vi "While_For_DIsplay-MSI.vi"() -> ()   [LabVIEW 2020]
panel:
  out "e 2":bool
  out "f 2":bool
  out "g 2":bool
  out "d 2":bool
  out "c 2":bool
  out "b 2":bool
  out "a 2":bool
  in  "stop":bool
  out "a":bool
  out "b":bool
  out "c":bool
  out "d":bool
  out "g":bool
  out "f":bool
  out "e":bool
  # "While"
  # "For"
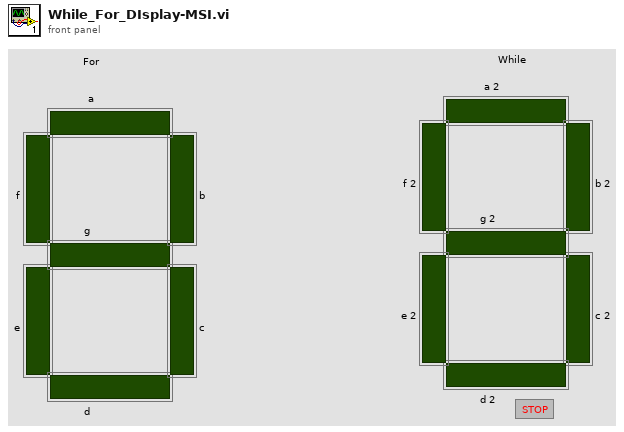
[diagram p1: front panel]
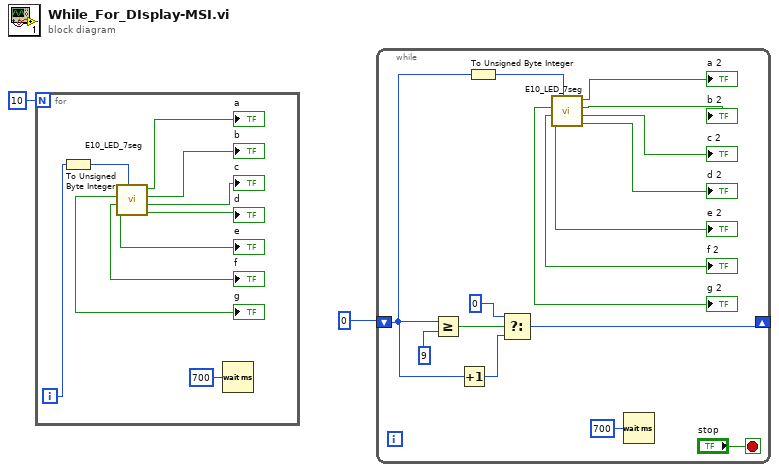
[diagram p0: block diagram]
diagram:
  n1 = for {
    N: 10 -> [_]
    i -> [w11]
    n2 = To Unsigned Byte Integer(number=w11) -> (unsigned 8bit integer=w10:u8)
    n3 = call "E10_LED_7seg.vi"("Numeric"=w10) -> ("d"=→"d":bool, "c"=→"c":bool, "b"=→"b":bool, "a"=→"a":bool, "e"=→"e":bool, "f"=→"f":bool, "g"=→"g":bool)  [unwired: 1 in]
    n4 = Wait (ms)(milliseconds to wait=u32 700) -> ()  [unwired: 1 out]
  }
  n5 = while {
    shift-right: [w20] -> _
    shift-left: 0 -> [w23]
    stop <- "stop" stop-if-true
    n6 = Greater Or Equal?(x=w23, y=9) -> (x >= y?=w24:bool)
    n7 = Increment(x=w23) -> (x+1=w22:i32)
    n8 = To Unsigned Byte Integer(number=w23) -> (unsigned 8bit integer=w28:u8)
    n9 = Select(t=0, s=w24, f=w22) -> (s? t:f=w20:i32)
    n10 = call "E10_LED_7seg.vi"("Numeric"=w28) -> ("d"=→"d 2":bool, "c"=→"c 2":bool, "b"=→"b 2":bool, "a"=→"a 2":bool, "e"=→"e 2":bool, "f"=→"f 2":bool, "g"=→"g 2":bool)  [unwired: 1 in]
    n11 = Wait (ms)(milliseconds to wait=u32 700) -> ()  [unwired: 1 out]
  }
